vi "Preview Waveform.vi"(4 "Decimation Multiple":u16, 8 "Channel #":i8, 9 "In Use?":bool, 10 "New Y Values":dbl[][](array[numeric]), 11 "Old Y Values":dbl[][](array[numeric])) -> (3 "Output Y Values":dbl[](array[numeric]))   [LabVIEW 2014]
panel:
  # "Preview Waveform"
  # "Inputs"
  # "Outputs"
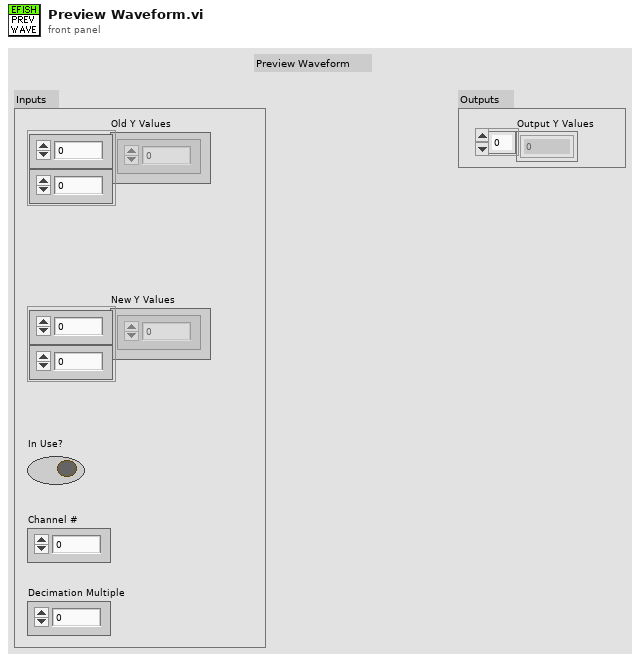
[diagram p1: front panel]
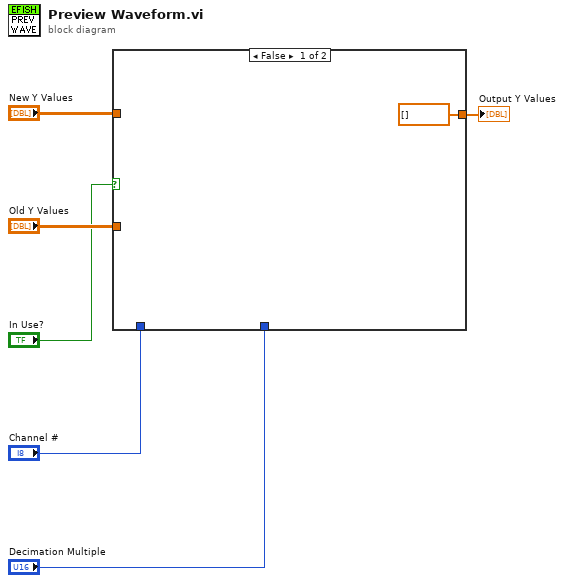
[diagram p0: block diagram]
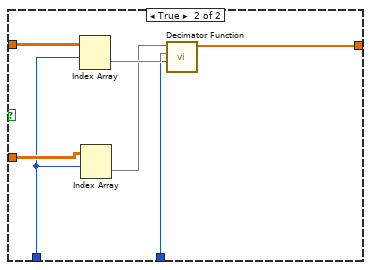
[diagram p2: hidden frame]
diagram:
  n1 = case shown="False" "In Use?" {
    tunnel: "New Y Values" -> [_ w14]
    tunnel: "Old Y Values" -> [_ w12]
    tunnel: "Channel #" -> [_ w11]
    tunnel: "Decimation Multiple" -> [_ w9]
    tunnel: [dbl[] [] ("Output Y Values") w8] -> w1
    frame False {
    }
    frame True {
      n2 = Index Array(array=w14, index (row)=w11) -> (element=w13:dbl[])  [unwired: 1 in]
      n3 = Index Array(array=w12, index (row)=w11) -> (element=w10:dbl[])  [unwired: 1 in]
      n4 = call "Decimator Function.vi"("Decimation #"=w9, "Input Y values New"=w13, "Input Y values Old"=w10) -> ("Output Y Values"=w8:dbl[])  [unwired: 8 in]
    }
  }
  "Output Y Values" <- w1
